vi "探头窗口-16.vi"() -> ()   [LabVIEW 2017]
panel:
  in  "更新数据":T1
  in  "停止信号":bool=TRUE
  out "更新数据？":bool=TRUE
  out "引用-切回列表模式？":refnum<vi>
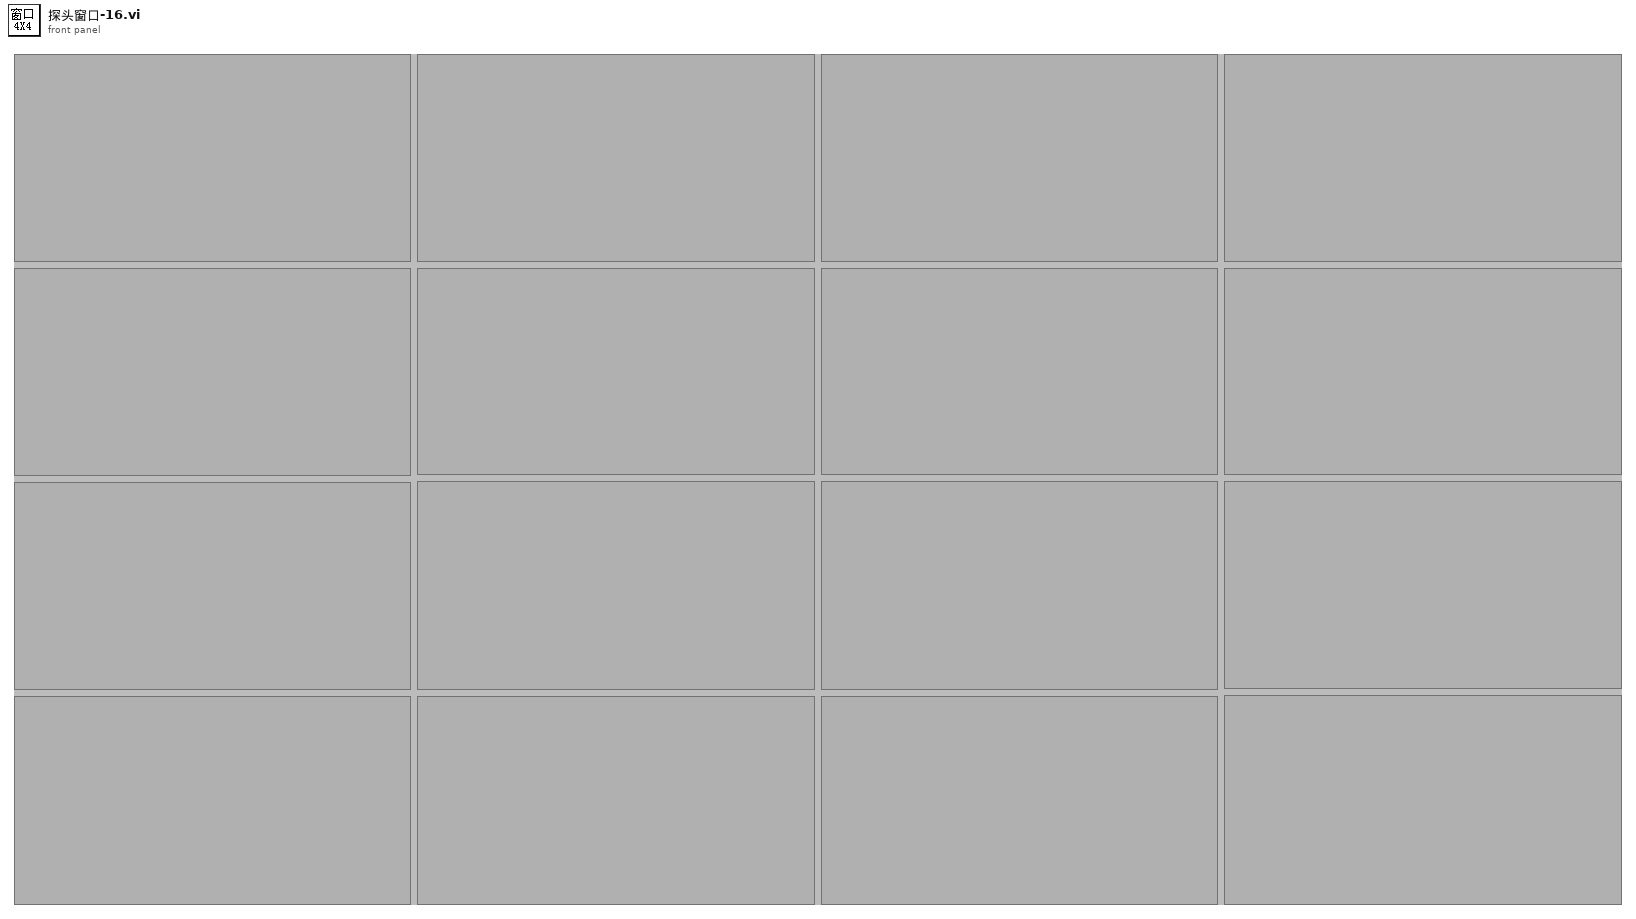
[diagram p1: front panel]
types:
  T1 = cluster{"探头启用状态？":bool[], "测量值":cluster{"X":timestamp, "Y":dbl}[], "限值":cluster{"限值1":dbl, "限值2":dbl, "探头限值":enum16{"一级限值", "二级限值"}}[], "报警状态":enum16{"正常", "一级报警", "二级报警", "累积报警"}[], "探头信息":string[], "累积剂量":cluster{"设备名称":string, "启用累积？":bool, "起始时间":timestamp, "累积剂量":dbl, "累积报警阈值":dbl}[]}
  T2 = cluster{"启用状态？":bool, "测量值":cluster{"X":timestamp, "Y":dbl}, "限值簇":cluster{"限值1":dbl, "限值2":dbl, "探头限值":enum16{"一级限值", "二级限值"}}, "报警状态":enum16{"正常", "一级报警", "二级报警", "累积报警"}, "探头信息":string, "探头地址":i32, "累积剂量":cluster{"设备名称":string, "启用累积？":bool, "起始时间":timestamp, "累积剂量":dbl, "累积报警阈值":dbl}}
  T3 = typedef "eventvkey.ctl" = enum16{"ASCII", "Enter", "Return", "Shift", "Ctrl", "Alt", "Cmd", "Opt", "Caps", "NumLock", "Clear", "Break", "Up", "Down", "Left", "Right", "Insert", "Delete", "Home", "End", "PageUp", "PageDown", "Escape", "Help", "Pause", "ScrollLock", "F1", "F2", "F3", "F4", "F5", "F6", "F7", "F8", "F9", "F10", "F11", "F12", "F13", "F14", "F15", "F16", "F17", "F18", "F19", "F20", "F21", "F22", "F23", "F24", "Play", "VolumeUp", "VolumeDown", "Mute", "Two Byte Char"}
  T4 = cluster{"限值1":dbl, "限值2":dbl, "探头限值":enum16{"一级限值", "二级限值"}}
  T5 = cluster{"限值1":dbl, "限值2":dbl, "探头限值":enum16{"一级限值", "二级限值"}}[]
  T6 = cluster{"设备名称":string, "启用累积？":bool, "起始时间":timestamp, "累积剂量":dbl, "累积报警阈值":dbl}[]
  T7 = cluster{"设备名称":string, "启用累积？":bool, "起始时间":timestamp, "累积剂量":dbl, "累积报警阈值":dbl}
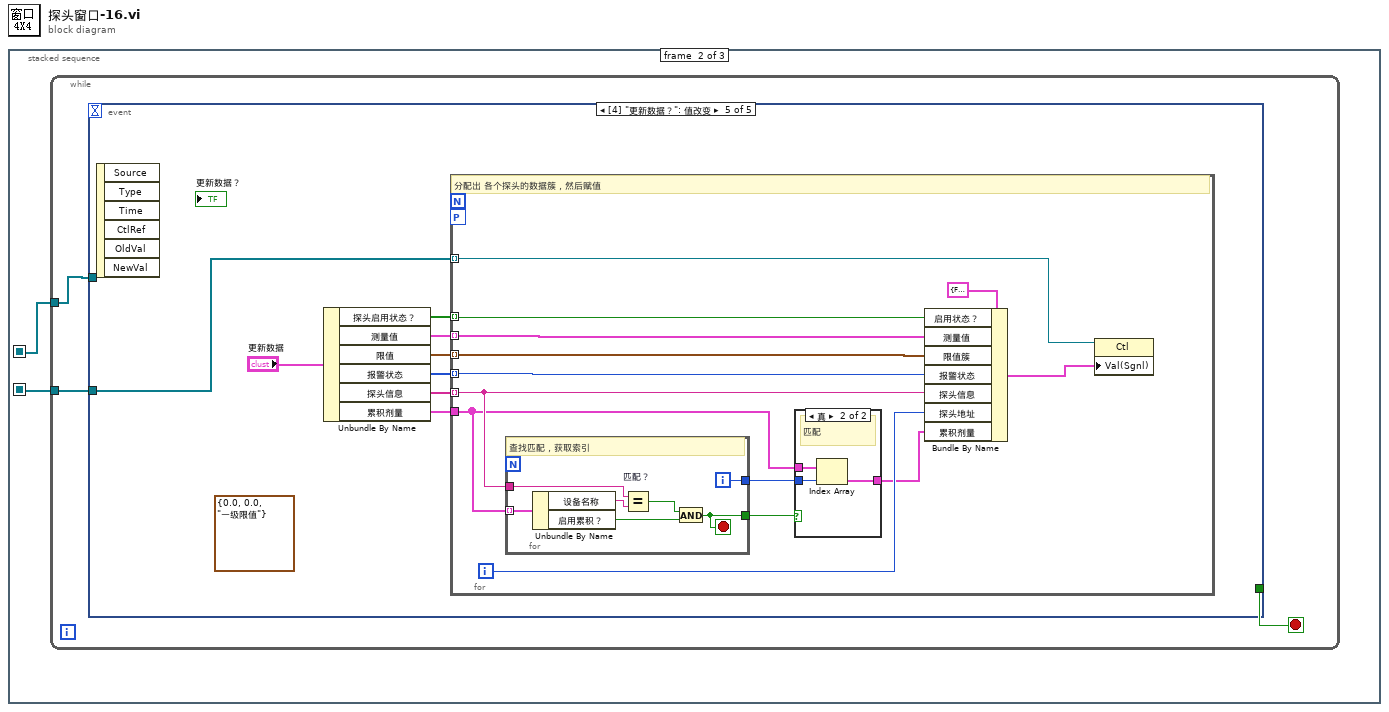
[diagram p0: block diagram]
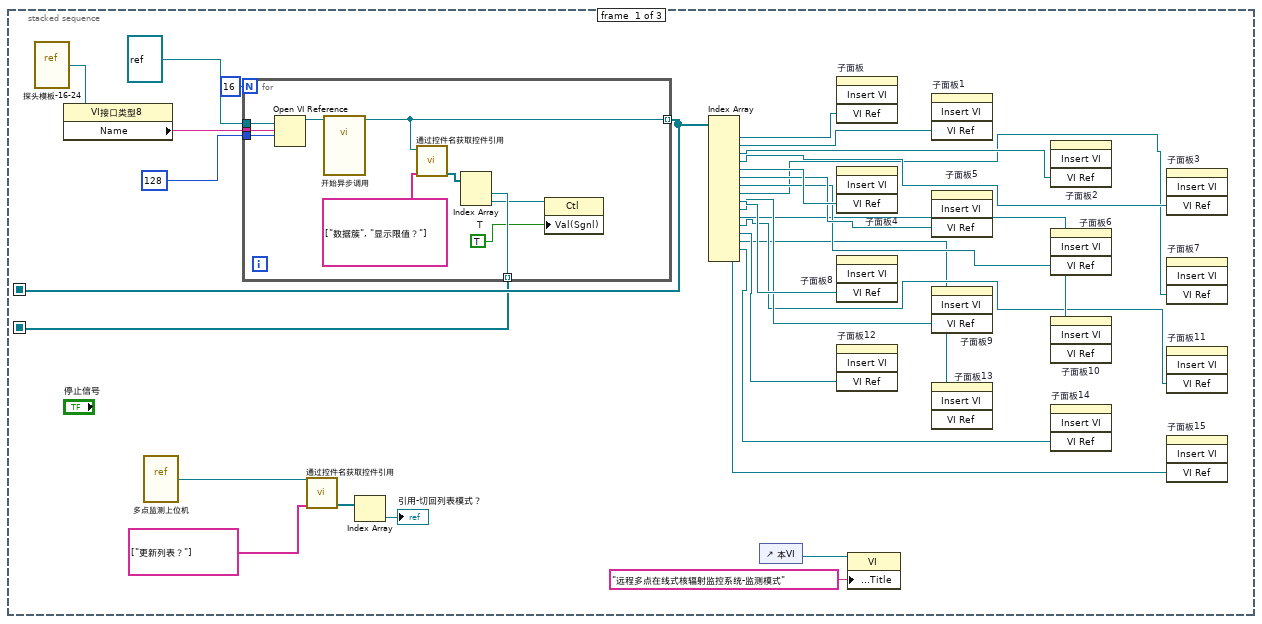
[diagram p2: hidden frame]
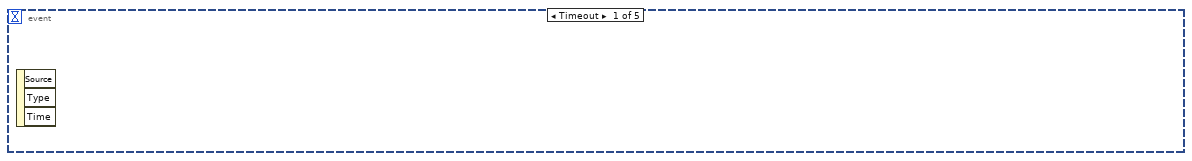
[diagram p3: hidden frame]
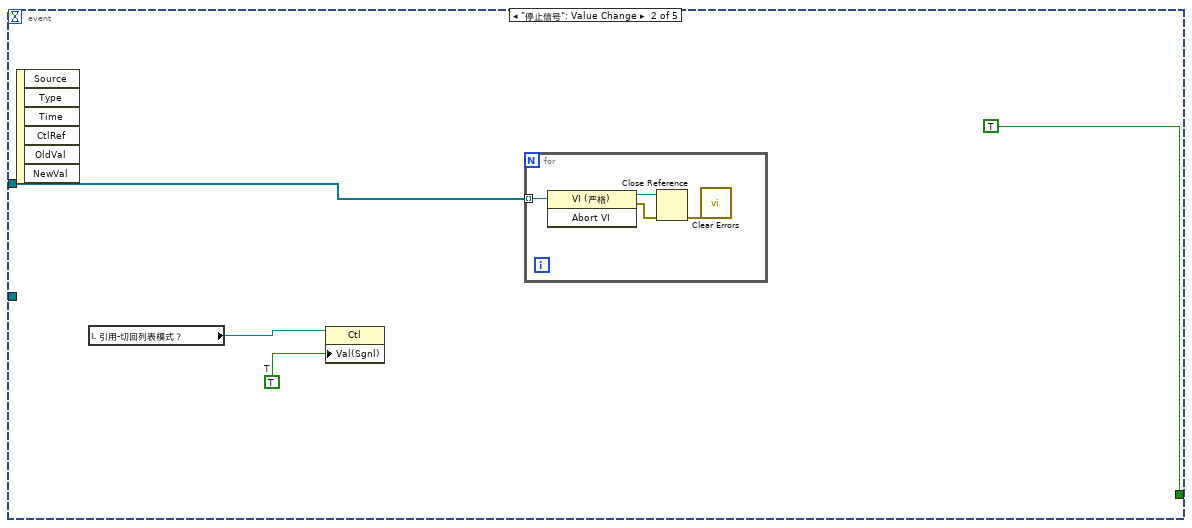
[diagram p4: hidden frame]
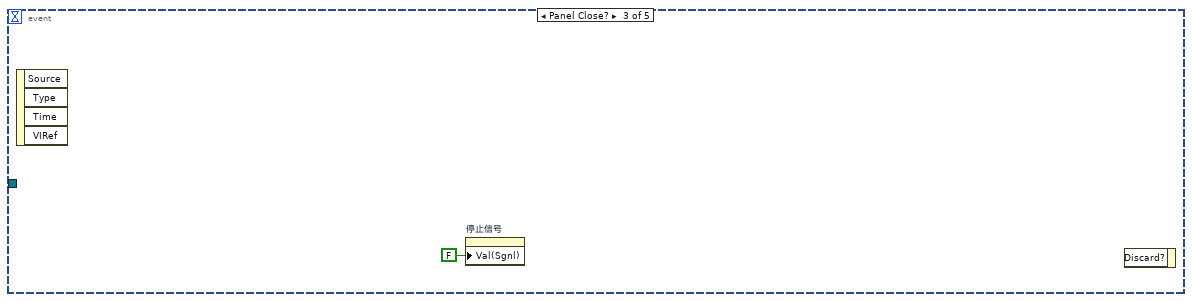
[diagram p5: hidden frame]
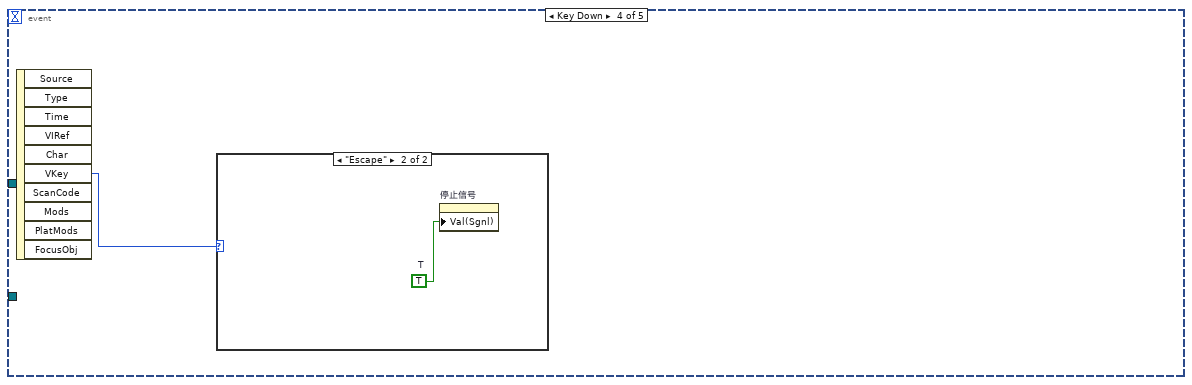
[diagram p6: hidden frame]
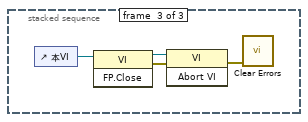
[diagram p9: hidden frame]
diagram:
  n1 = stacked-sequence {
    seq-local: [w24 _ _] -> [_ w41 _]
    seq-local: [w3 _ _] -> [_ w40 _]
    frame #0 {
      n2 = vi-ref "探头模板-16-24.vi"() -> (w29:refnum<vi>)
      n3 = property class="VI接口类型8"(reference=w29) -> ("Name"=w28:string)  [unwired: 1 in, 2 out]
      n4 = vi-ref "多点监测上位机.vi"() -> (w4:refnum<vi>)
      n5 = for {
        N: 16 -> [_]
        tunnel: w28 -> [w39]
        tunnel: 128 ("选项") -> [w38]
        tunnel: refnum<vi> refnum ("类型说明符VI引用句柄（仅用于类型）") -> [w37]
        tunnel: [w32] -> w24 mode=indexing
        tunnel: [w33] -> w3 mode=indexing
        w30 = TRUE  # T
        n6 = Open VI Reference(type specifier VI Refnum (for type only)=w37, vi path=w39, options=w38) -> (vi reference=w34:refnum<vi>)  [unwired: 3 in, 1 out]
        n7 = call-by-ref "开始异步调用"(reference=w34) -> (reference out=w32:refnum<vi>)  [unwired: 13 in, 1 out]
        n8 = call "通过控件名获取控件引用.vi"("控件名数组"=string[] ["数据簇", "显示限值？"], "VI引用"=w32) -> ("控件引用输出"=w36:refnum<vi>[])  [unwired: 7 in, 2 out]
        n9 = Index Array(array=w36) -> (element #1=w33:refnum<vi>, element #2=w31:refnum<vi>)  [unwired: 2 in]
        n10 = property class="Ctl"(reference=w31, "Val(Sgnl)"=w30) -> ()  [unwired: 1 in, 2 out]
      }
      n11 = call "通过控件名获取控件引用.vi"("控件名数组"=string[] ["更新列表？"], "VI引用"=w4) -> ("控件引用输出"=w6:refnum<vi>[])  [unwired: 7 in, 2 out]
      n12 = Index Array(array=w6) -> (element=→"引用-切回列表模式？":refnum<vi>)  [unwired: 1 in]
      n13 = Index Array(array=w24) -> (element #1=w23:refnum<vi>, element #2=w22:refnum<vi>, element #3=w21:refnum<vi>, element #4=w20:refnum<vi>, element #5=w19:refnum<vi>, element #6=w18:refnum<vi>, element #7=w17:refnum<vi>, element #8=w16:refnum<vi>, element #9=w15:refnum<vi>, element #10=w14:refnum<vi>, element #11=w13:refnum<vi>, element #12=w12:refnum<vi>, element #13=w11:refnum<vi>, element #14=w10:refnum<vi>, element #15=w9:refnum<vi>, element #16=w8:refnum<vi>)  [unwired: 16 in]
      n14 = control-ref of="本VI"() -> (w2:refnum<vi>)
      n15 = invoke on="子面板" class="子面板" method="Insert VI"("VI Ref"=w23) -> ()  [unwired: 3 in, 4 out]
      n16 = invoke on="子面板4" class="SubPnl" method="Insert VI"("VI Ref"=w19) -> ()  [unwired: 3 in, 4 out]
      n17 = invoke on="子面板8" class="SubPnl" method="Insert VI"("VI Ref"=w15) -> ()  [unwired: 3 in, 4 out]
      n18 = invoke on="子面板12" class="SubPnl" method="Insert VI"("VI Ref"=w11) -> ()  [unwired: 3 in, 4 out]
      n19 = property class="VI"(reference=w2, "Front Panel.Title"="远程多点在线式核辐射监控系统-监测模式" ("前面板窗口:标题")) -> ()  [unwired: 1 in, 2 out]
      n20 = invoke on="子面板1" class="SubPnl" method="Insert VI"("VI Ref"=w22) -> ()  [unwired: 3 in, 4 out]
      n21 = invoke on="子面板5" class="SubPnl" method="Insert VI"("VI Ref"=w18) -> ()  [unwired: 3 in, 4 out]
      n22 = invoke on="子面板9" class="SubPnl" method="Insert VI"("VI Ref"=w14) -> ()  [unwired: 3 in, 4 out]
      n23 = invoke on="子面板13" class="SubPnl" method="Insert VI"("VI Ref"=w10) -> ()  [unwired: 3 in, 4 out]
      n24 = invoke on="子面板2" class="SubPnl" method="Insert VI"("VI Ref"=w21) -> ()  [unwired: 3 in, 4 out]
      n25 = invoke on="子面板6" class="SubPnl" method="Insert VI"("VI Ref"=w17) -> ()  [unwired: 3 in, 4 out]
      n26 = invoke on="子面板10" class="SubPnl" method="Insert VI"("VI Ref"=w13) -> ()  [unwired: 3 in, 4 out]
      n27 = invoke on="子面板14" class="SubPnl" method="Insert VI"("VI Ref"=w9) -> ()  [unwired: 3 in, 4 out]
      n28 = invoke on="子面板3" class="SubPnl" method="Insert VI"("VI Ref"=w20) -> ()  [unwired: 3 in, 4 out]
      n29 = invoke on="子面板7" class="SubPnl" method="Insert VI"("VI Ref"=w16) -> ()  [unwired: 3 in, 4 out]
      n30 = invoke on="子面板11" class="SubPnl" method="Insert VI"("VI Ref"=w12) -> ()  [unwired: 3 in, 4 out]
      n31 = invoke on="子面板15" class="SubPnl" method="Insert VI"("VI Ref"=w8) -> ()  [unwired: 3 in, 4 out]
    }
    frame #1 {
      n32 = while {
        tunnel: w41 -> [w43]
        tunnel: w40 -> [w42]
        stop <- w44 stop-if-true
        n33 = event shown="[4] \"更新数据？\": 值改变" {
          selector: _ -> [_ _ _ _ _]
          dyn-events: _ -> [_ _ _ _ _]
          timeout: _ -> [_ _ _ _ _]
          tunnel: [_ TRUE ("放弃？") _ _ _] -> w44
          tunnel: w43 -> [_ w47 _ _ _]
          tunnel: w42 -> [_ _ _ _ w56]
          event Timeout {
            n34 = event-data() -> ()  [unwired: 1 in, 3 out]
          }
          event "停止信号": Value Change {
            w46 = TRUE  # T
            n35 = event-data() -> ()  [unwired: 1 in, 6 out]
            n36 = local read "引用-切回列表模式？"() -> (w45:refnum<vi>)
            n37 = property class="Ctl"(reference=w45, "Val(Sgnl)"=w46) -> ()  [unwired: 1 in, 2 out]
            n38 = for {
              tunnel: w47 -> [w52] mode=indexing
              n39 = invoke class="VI (严格)" method="Abort VI"(reference=w52) -> (reference out=w50:refnum<vi>, error out=w51:errorcluster)  [unwired: 2 in, 1 out]
              n40 = Close Reference(reference=w50, error in (no error)=w51) -> (error out=w49:errorcluster)
              n41 = call <vilib>:"Clear Errors.vi"("error in (no error)"=w49) -> ()  [unwired: 5 in, 2 out]
            }
          }
          event Panel Close? {
            n42 = event-data() -> ()  [unwired: 1 in, 4 out]
            n43 = property on="停止信号" class="Bool (严格)"("Val(Sgnl)"=FALSE ("值(信号)")) -> ()  [unwired: 2 in, 2 out]
            n44 = event-data() -> ()  [unwired: 2 in, 1 out]
          }
          event Key Down {
            n45 = event-data() -> ("VKey"=w54:T3)  [unwired: 1 in, 9 out]
            n46 = case shown="\"Escape\"" w54 {
              frame "ASCII", Default {
              }
              frame "Escape" {
                w55 = TRUE  # T
                n47 = property on="停止信号" class="Bool (严格)"("Val(Sgnl)"=w55) -> ()  [unwired: 2 in, 2 out]
              }
            }
          }
          event "更新数据？": Value Change {
            (unwired) T4 {"限值1"=0.0, "限值2"=0.0, "探头限值"=enum."一级限值"} ("探头限值簇")
            n48 = event-data() -> ()  [unwired: 1 in, 6 out]
            n49 = Unbundle By Name("更新数据") -> ("探头启用状态？"=w57:bool[], "测量值"=w58:cluster{"X":timestamp, "Y":dbl}[], "限值"=w59:T5, "报警状态"=w60:enum16{"正常", "一级报警", "二级报警", "累积报警"}[], "探头信息"=w61:string[], "累积剂量"=w62:T6)
            n50 = for {
              tunnel: w57 -> [w76] mode=indexing
              tunnel: w58 -> [w75] mode=indexing
              tunnel: w59 -> [w74] mode=indexing
              tunnel: w60 -> [w73] mode=indexing
              tunnel: w61 -> [w68] mode=indexing
              workers-P: _ -> [_]
              tunnel: w56 -> [w71] mode=indexing
              tunnel: w62 -> [w67]
              i -> [w69]
              # "分配出 各个探头的数据簇，然后赋值"
              n51 = for {
                tunnel: w67 -> [w86] mode=indexing
                tunnel: w68 -> [w84]
                tunnel: [w81] -> w66
                tunnel: [w80] -> w65
                i -> [w81]
                stop <- w80 stop-if-true
                # "查找匹配，获取索引"
                n52 = Unbundle By Name(w86) -> ("设备名称"=w85:string, "启用累积？"=w82:bool)
                n53 = Equal? "匹配？"(x=w84, y=w85) -> (x = y?=w83:bool)
                n54 = And(x=w83, y=w82) -> (x .and. y?=w80:bool)
              }
              n55 = case shown="真" w65 {
                tunnel: w67 -> [_ w79]
                tunnel: w66 -> [_ w78]
                tunnel: [_ w77] -> w64
                frame False {
                  # "不匹配"
                }
                frame True {
                  # "匹配"
                  n56 = Index Array(array=w79, index=w78) -> (element=w77:T7)
                }
              }
              n57 = Bundle By Name(cluster=T2 {"启用状态？"=FALSE, "测量值"={"X"=timestamp(0 s since 1904-01-01), "Y"=0.0}, "限值簇"={"限值1"=0.0, "限值2"=0.0, "探头限值"=enum."一级限值"}, "报警状态"=enum."正常", "探头信息"="", "探头地址"=0, "累积剂量"={"设备名称"="", "启用累积？"=FALSE, "起始时间"=timestamp(0 s since 1904-01-01), "累积剂量"=0.0, "累积报警阈值"=0.0}} ("输出簇"), "启用状态？"=w76, "测量值"=w75, "限值簇"=w74, "报警状态"=w73, "探头信息"=w68, "探头地址"=w69, "累积剂量"=w64) -> (w70:T2)
              n58 = property class="Ctl"(reference=w71, "Val(Sgnl)"=w70) -> ()  [unwired: 1 in, 2 out]
            }
          }
        }
      }
    }
    frame #2 {
      n59 = control-ref of="本VI"() -> (w90:refnum<vi>)
      n60 = invoke class="VI" method="FP.Close"(reference=w90) -> (reference out=w89:refnum<vi>, error out=w88:errorcluster)  [unwired: 2 in, 1 out]
      n61 = invoke class="VI" method="Abort VI"(reference=w89, error in=w88) -> (error out=w87:errorcluster)  [unwired: 1 in, 2 out]
      n62 = call <vilib>:"Clear Errors.vi"("error in (no error)"=w87) -> ()  [unwired: 5 in, 2 out]
    }
  }
